vi "test Find One Frame.vi"(8 "error in (no error)":errorcluster, 11 "TestCase in":refnum<class "Test Find Complete Frame.lvclass">) -> (0 "error out":errorcluster, 3 "TestCase out":refnum<class "Test Find Complete Frame.lvclass">)   [LabVIEW 2018, in "Test Find Complete Frame.lvclass"]
uses:
  Test Find Complete Frame.lvclass
  Libraries/iTacho_class/iTacho.lvclass
  <vilib>/addons/_JKI Toolkits/VI Tester/TestCase.llb/TestCase.lvclass
  C:/Program Files (x86)/National Instruments/LabVIEW 2018/vi.lib/addons/_JKI Toolkits/VI Tester/TestCase.llb/TestCase.lvclass
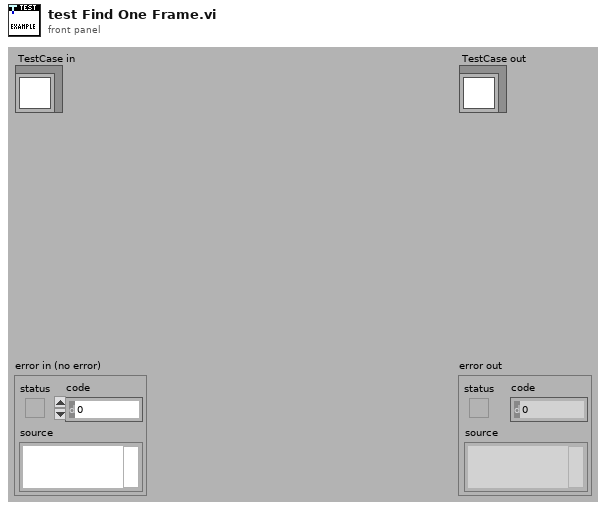
[diagram p1: front panel]
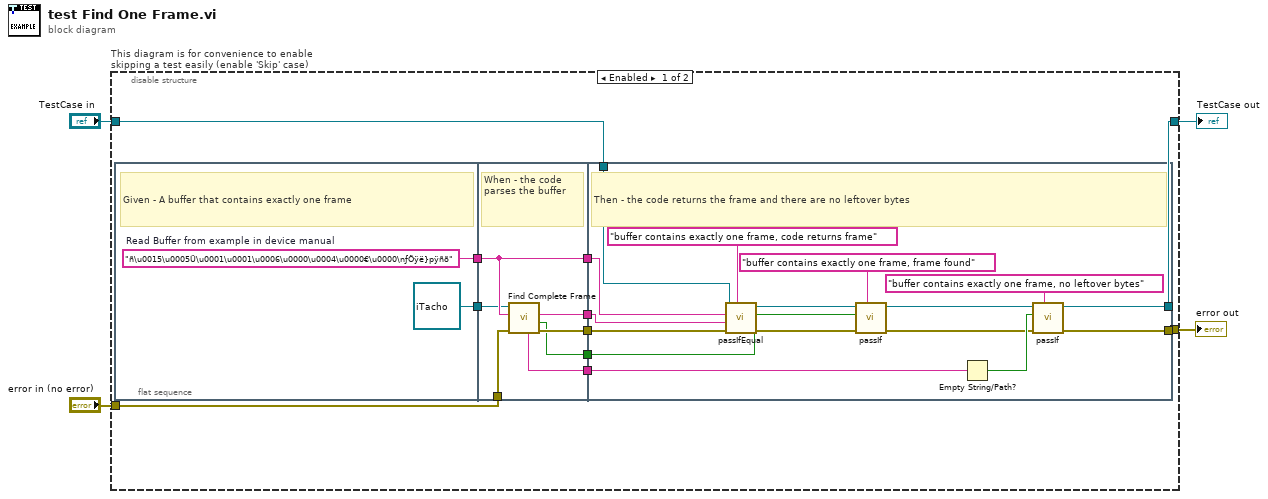
[diagram p0: block diagram]
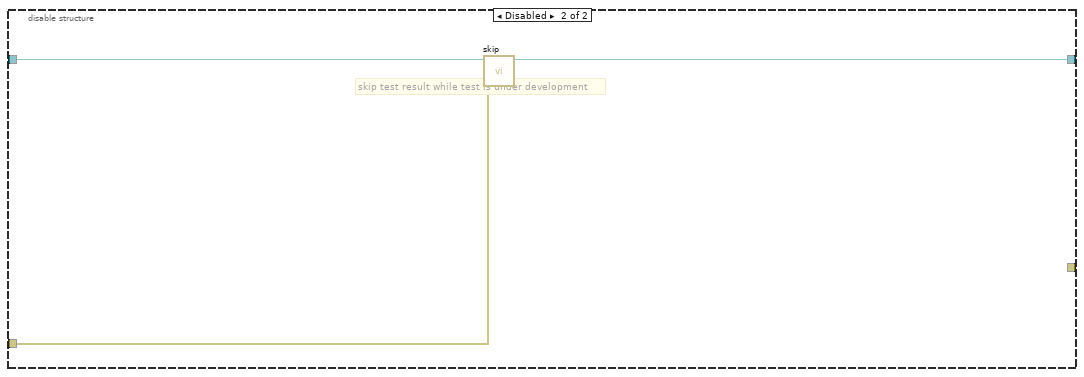
[diagram p2: hidden frame]
diagram:
  n1 = disable-structure "This diagram is for convenience to enable skipping a test easily (enable 'Skip' case)" shown="Enabled" {
    disable-tunnel: "TestCase in" -> [w6 w44]
    disable-tunnel: [w5 w42] -> w1
    disable-tunnel: "error in (no error)" -> [w9 w41]
    disable-tunnel: [w7 _] -> w2
    frame Enabled {
      n2 = flat-sequence {
        tunnel: [refnum<class "iTacho.lvclass"> refnum ("iTacho in")] -> w15
        tunnel: [w16] -> w14
        tunnel: w15 -> [w22]
        tunnel: w14 -> [w23]
        tunnel: [w23] -> w13
        tunnel: [w21] -> w12
        tunnel: [w20] -> w11
        tunnel: [w19] -> w10
        tunnel: w9 -> [w18]
        tunnel: [w24] -> w8
        tunnel: w13 -> [w36]
        tunnel: w12 -> [w33]
        tunnel: w11 -> [w35]
        tunnel: w10 -> [w40]
        tunnel: w8 -> [w38]
        tunnel: w6 -> [w37]
        tunnel: [w28] -> w7
        tunnel: [w27] -> w5
        frame #0 {
          w16 = "ñ\u0015\u0005Ü\u0001\u0001\u0006\u0000\u0004\u0000€\u0000\nƒÖÿë}pÿñõ"  # Read Buffer from example in device manual
          # "Given - A buffer that contains exactly one frame"
        }
        frame #1 {
          # "When - the code parses the buffer"
          n3 = call-dynamic "Find Complete Frame.vi"("error in (no error)"=w18, "Read Buffer in"=w23, "iTacho in"=w22) -> ("error out"=w24:errorcluster, "Found New Frame?"=w21:bool, "Frame"=w20:string, "Leftover Bytes"=w19:string)  [unwired: 4 in, 1 out]
        }
        frame #2 {
          # "Then - the code returns the frame and there are no leftover bytes"
          n4 = call-dynamic "passIfEqual.vi"("custom report message (\"\")"="buffer contains exactly one frame, code returns frame" ("custom report message (\"\")"), "error in (no error)"=w38, "y"=w35, "x"=w36, "TestCase in"=w37) -> ("error out"=w31:errorcluster, "TestCase out"=w32:refnum<class "Test Find Complete Frame.lvclass">)  [unwired: 5 in]
          n5 = call-dynamic "passIf.vi"("custom report message (\"\")"="buffer contains exactly one frame, frame found" ("custom report message (\"\")"), "error in (no error)"=w31, "pass"=w33, "TestCase in"=w32) -> ("error out"=w29:errorcluster, "TestCase out"=w30:refnum<class "Test Find Complete Frame.lvclass">)  [unwired: 6 in]
          n6 = Empty String/Path?(string/path=w40) -> (empty?=w34:bool)
          n7 = call-dynamic "passIf.vi"("custom report message (\"\")"="buffer contains exactly one frame, no leftover bytes" ("custom report message (\"\")"), "error in (no error)"=w29, "pass"=w34, "TestCase in"=w30) -> ("error out"=w28:errorcluster, "TestCase out"=w27:refnum<class "Test Find Complete Frame.lvclass">)  [unwired: 6 in]
        }
      }
    }
    frame Disabled {
      # "skip test result while test is under development"
      n8 = call <vilib>:"skip.vi"("error in (no error)"=w41, "TestCase in"=w44) -> ("error out"=w43:errorcluster, "TestCase out"=w42:refnum<class "Test Find Complete Frame.lvclass">)  [unwired: 8 in]
    }
  }
  "error out" <- w2
  "TestCase out" <- w1
